vi "Vars_Init.vi"(9 "Data Cluster In":T1, 10 "Init? In":bool, 11 "WriteVars?":bool) -> (1 "Data Cluster Out":T1, 2 "Init? Out":bool)   [LabVIEW 2014]
uses:
  type_def/DataCluster.ctl
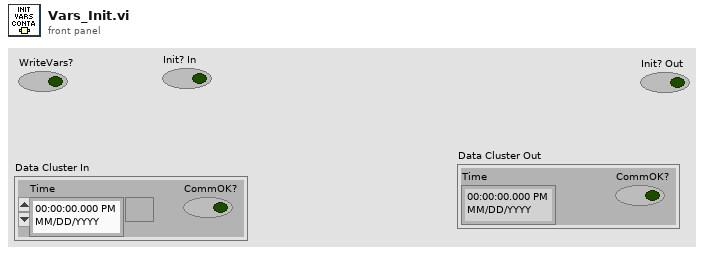
[diagram p1: front panel]
types:
  T1 = typedef "DataCluster.ctl" = cluster{"Time":timestamp, "CommOK?":bool}
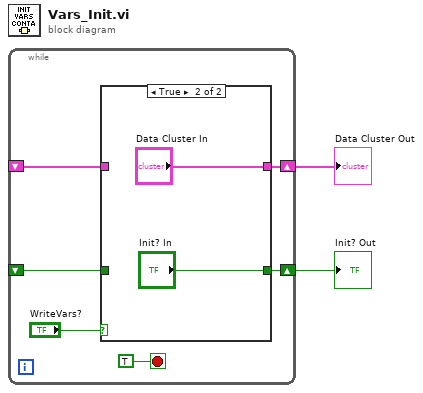
[diagram p0: block diagram]
diagram:
  n1 = while {
    shift-right: [w6] -> w2
    shift-left: _ -> [w4]
    shift-right: [w5] -> w1
    shift-left: _ -> [w3]
    stop <- TRUE stop-if-true
    n2 = case shown="True" "WriteVars?" {
      tunnel: [w10 "Data Cluster In"] -> w6
      tunnel: [w9 "Init? In"] -> w5
      tunnel: w4 -> [w10 _]
      tunnel: w3 -> [w9 _]
      frame False {
      }
      frame True {
      }
    }
  }
  "Init? Out" <- w1
  "Data Cluster Out" <- w2
